vi "BIO_set_accept_BIOs.vi"(8 "error in (no error)":errorcluster, 10 "SSL BIO":refnum<class "BIO.lvclass">, 11 "Accept BIO in":refnum<class "BIO.lvclass">) -> (0 "error out":errorcluster, 3 "Accept BIO out":refnum<class "BIO.lvclass">)   [LabVIEW 2013, in "SSL_Lib.lvlib" / "BIO.lvclass"]
uses:
  BIO.lvclass
  SSL-Lib/SSL-Lib.lvclass/SSL-Lib.ctl
  BIO.lvclass/BIO.ctl
  Read Handle.vi
  SSL-Lib/Read Crypto Library Path.vi
  SSL-Lib/SSL-Lib.lvclass
panel:
  out "return type":i32
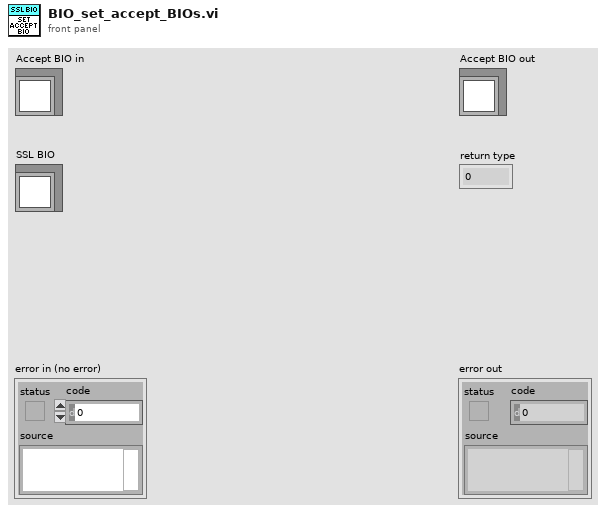
[diagram p1: front panel]
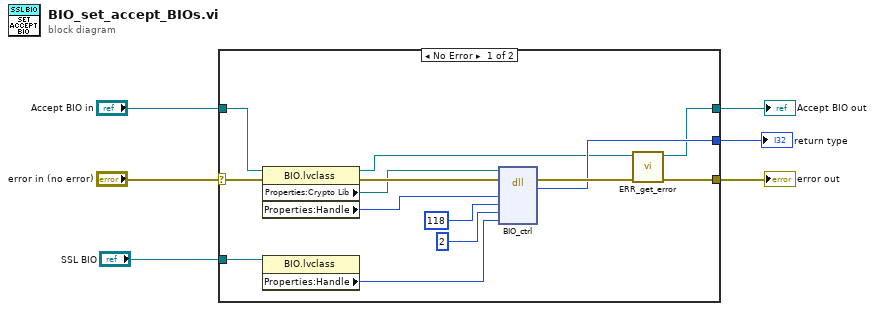
[diagram p0: block diagram]
diagram:
  n1 = case shown="No Error" "error in (no error)" {
    selector: "error in (no error)" -> [w20 w22]
    tunnel: [w10 w22] -> w5
    tunnel: [w8 w21] -> w3
    tunnel: "Accept BIO in" -> [w15 w21]
    tunnel: [w17 _] -> w2
    tunnel: "SSL BIO" -> [w12 _]
    frame No Error {
      n2 = property class="BIO.lvclass"(reference=w15, error in=w20) -> (reference out=w9:refnum<class "BIO.lvclass">, error out=w16:errorcluster, "Properties:Crypto Lib"=w14:path, "Properties:Handle"=w13:u64)
      n3 = property class="BIO.lvclass"(reference=w12) -> ("Properties:Handle"=w11:u64)  [unwired: 1 in, 2 out]
      n4 = dll-call lib="C:/Program Files (x86)/National Instruments/Shared/nissl/NIssleay32.dll" fn="BIO_ctrl"(path in=w14, error in=w16, "BIO"=w13, "cmd"=118, "larg"=2, "parg"=w11) -> (error out=w19:errorcluster, "return type"=w17:i32)  [unwired: 5 in, 1 out]
      n5 = call "ERR_get_error.vi"("error in (no error)"=w19, "SSL-Lib in"=w9) -> ("error out"=w10:errorcluster, "SSL-Lib out"=w8:refnum<class "BIO.lvclass">)  [unwired: 8 in]
    }
    frame Error {
    }
  }
  "error out" <- w5
  "Accept BIO out" <- w3
  "return type" <- w2
